vi "MT -Move to hardware travel limit.vi"(7 "Action":bool, 8 "error in":errorcluster, 9 "Move to travel limit\nset (+ or - )":dbl format="%.2f", 10 "Axis #":i8=1 min=1 max=6 step=1, 11 "Address / Port":i16=1 min=1 max=31 step=1) -> (0 "error out":errorcluster, 1 "Motion Status\nread":string, 2 "Axis out":i8=1 min=1 max=6 step=1, 3 "Address / Port out":i16=1 min=1 max=31 step=1)   [LabVIEW 2014]
panel:
  # "Read"
  # "Write"
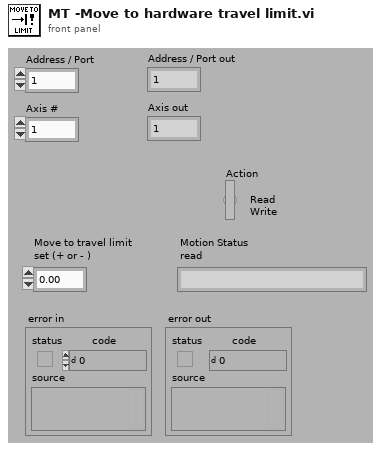
[diagram p1: front panel]
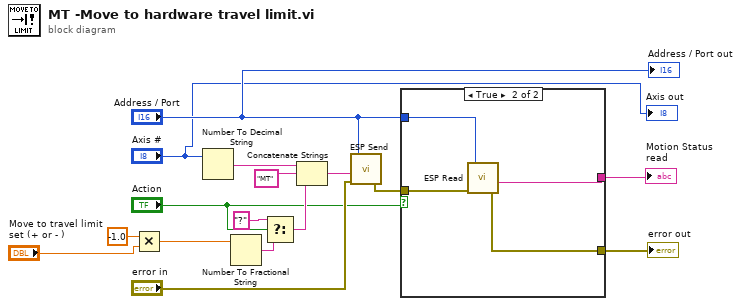
[diagram p0: block diagram]
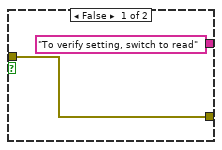
[diagram p2: hidden frame]
diagram:
  n1 = Multiply(x=-1.0, y="Move to travel limit\nset (+ or - )") -> (x*y=w1:dbl)
  n2 = Number To Decimal String(number="Axis #") -> (decimal integer string=w16:string)  [unwired: 1 in]
  n3 = Number To Fractional String(number=w1) -> (F-format string=w12:string)  [unwired: 3 in]
  n4 = Select(t="?", s="Action", f=w12) -> (s? t:f=w13:string)
  n5 = Concatenate Strings(w16, "MT" ("Substring"), w13) -> (w14:string)
  n6 = call "ESP Send.vi"("error in"="error in", "Command String"=w14, "Address / Port"="Address / Port") -> ("error out"=w8:errorcluster)  [unwired: 3 in, 1 out]
  n7 = case shown="True" "Action" {
    tunnel: "Address / Port" -> [_ w22]
    tunnel: w8 -> [w18 w21]
    tunnel: [w18 w20] -> w7
    tunnel: ["To verify setting, switch to read" w19] -> w6
    frame False {
    }
    frame True {
      n8 = call "ESP Read.vi"("error in"=w21, "Address / Port"=w22) -> ("error out"=w20:errorcluster, "Response String"=w19:string)  [unwired: 3 in, 1 out]
    }
  }
  "error out" <- w7
  "Motion Status\nread" <- w6
  "Address / Port out" <- "Address / Port"
  "Axis out" <- "Axis #"
